vi "百分比.vi"(8 "已发帧数 2":i32, 9 "发第几次":i32, 10 "帧数":i32, 11 "共发送次数":string) -> (1 "已发送百分比":u8, 2 "已传百分比":string)   [LabVIEW 2016, in "数据传输系统.lvlib" / "自动更新.lvlib" / "TCP文件传输系统.lvlib" / "TCP发送文件.lvlib"]
panel:
  out "在发第几次":i32
  out "共发送次数":string
  out "侦数":i32
  out "已发帧数":i32
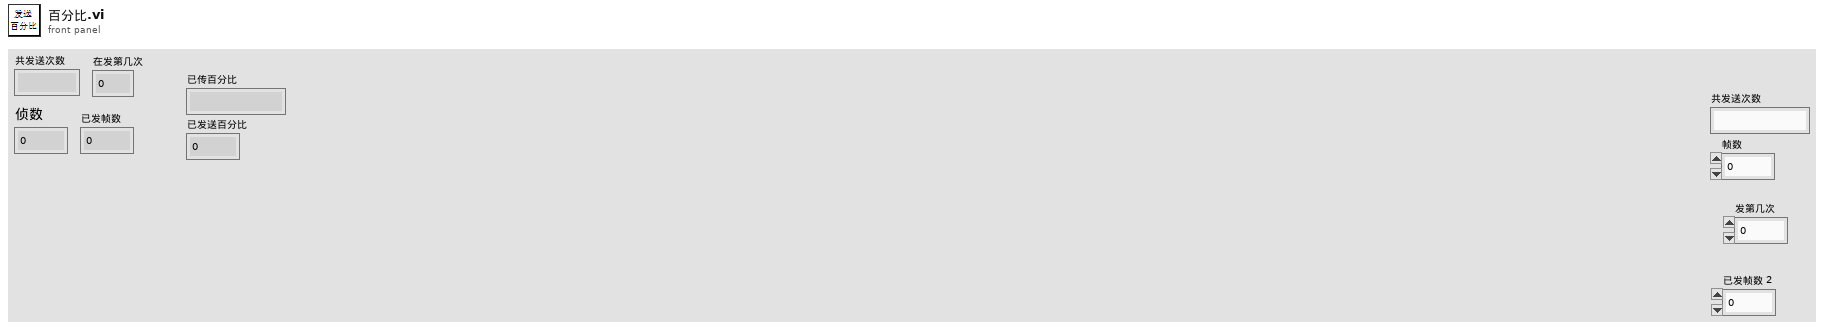
[diagram p1: front panel]
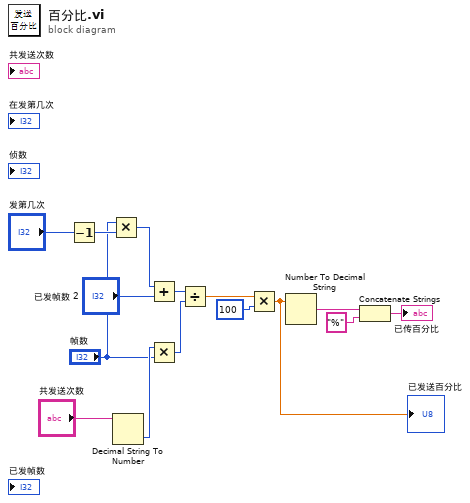
[diagram p0: block diagram]
diagram:
  n1 = Decrement(x="发第几次") -> (x-1=w10:i32)
  n2 = Multiply(x="帧数", y=w10) -> (x*y=w14:i32)
  n3 = Decimal String To Number(string="共发送次数") -> (number=w15:i32)  [unwired: 2 in, 1 out]
  n4 = Add(x=w14, y="已发帧数 2") -> (x+y=w7:i32)
  n5 = Multiply(x=w15, y="帧数") -> (x*y=w6:i32)
  n6 = Divide(x=w7, y=w6) -> (x/y=w5:dbl)
  n7 = Multiply(x=w5, y=100) -> (x*y=w9:dbl)
  "已发送百分比" <- w9
  n8 = Number To Decimal String(number=w9) -> (decimal integer string=w13:string)  [unwired: 1 in]
  n9 = Concatenate Strings(w13, "%" ("字符串")) -> (→"已传百分比":string)
